vi "Configure Component Values.vi"(0 "VISA resource name":refnum<visa-resource-name>, 1 "Relative Phase":bool, 5 "Frequency (10.000000 MHz)":dbl=10.0, 7 "Unit (MHz)":u16(ring)=1 items=["GHz", "MHz", "KHz", "Hz"], 9 "Phase (0°)":i32, 11 "error in (no error)":errorcluster) -> (4 "VISA resource name out":refnum<visa-resource-name>, 15 "error out":errorcluster)   [LabVIEW 2013, in "Stanford Research CG635.lvlib"]
doc: "Configures the <b>frequency</b> and the <b>phase</b> components to the specified values. \n\n<b>Ranges</b>\nFrequency: 1 µHz to 2.05 GHz\nPhase: -720° to 720°"
uses:
  <instrlib>/Stanford Research CG635/Stanford Research CG635.lvlib
panel:
  # "Note: Set's the current Phase to be a new realtive 0°"
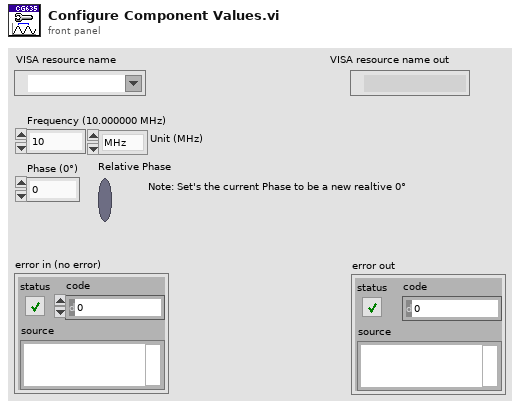
[diagram p1: front panel]
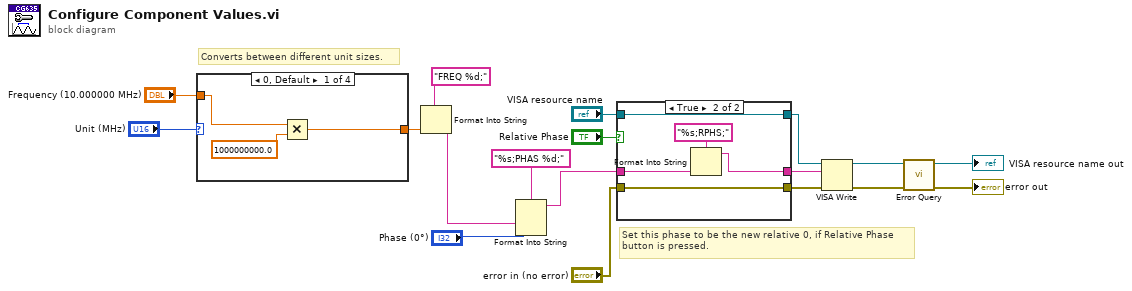
[diagram p0: block diagram]
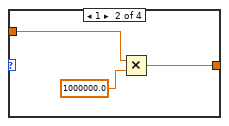
[diagram p3: hidden frame]
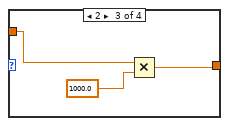
[diagram p4: hidden frame]
diagram:
  # "Set this phase to be the new relative 0, if Relative Phase \nbutton is pressed."
  # "Converts between different unit sizes."
  n1 = case shown="0, Default" "Unit (MHz)" {
    tunnel: "Frequency (10.000000 MHz)" -> [w21 w23 w25 w28]
    tunnel: [w19 w22 w26 w28] -> w13
    frame 0, Default {
      n2 = Multiply(x=w21, y=1000000000.0) -> (x*y=w19:dbl)
    }
    frame 1 {
      n3 = Multiply(x=w23, y=1000000.0) -> (x*y=w22:dbl)
    }
    frame 2 {
      n4 = Multiply(x=w25, y=1000.0) -> (x*y=w26:dbl)
    }
    frame 3 {
    }
  }
  n5 = Format Into String(format string="FREQ %d;", w13) -> (resulting string=w11:string)  [unwired: 2 in, 1 out]
  n6 = Format Into String(format string="%s;PHAS %d;", w11, "Phase (0°)") -> (resulting string=w8:string)  [unwired: 2 in, 1 out]
  n7 = case shown="True" "Relative Phase" {
    tunnel: [w29 w35] -> w12
    tunnel: w8 -> [w29 w34]
    tunnel: "VISA resource name" -> [w31 w33]
    tunnel: [w31 w33] -> w9
    tunnel: "error in (no error)" -> [w30 w32]
    tunnel: [w30 w32] -> w6
    frame False {
    }
    frame True {
      n8 = Format Into String(format string="%s;RPHS;", w34) -> (resulting string=w35:string)  [unwired: 2 in, 1 out]
    }
  }
  n9 = VISA Write(VISA resource name=w9, write buffer=w12, error in (no error)=w6) -> (VISA resource name out=w4:refnum<visa-resource-name>, error out=w3:errorcluster)  [unwired: 1 out]
  n10 = call <instrlib>:"Error Query.vi"("error in (no error)"=w3, "VISA resource name"=w4) -> ("error out"=→"error out":errorcluster, "VISA resource name out"=→"VISA resource name out":refnum<visa-resource-name>)  [unwired: 6 in, 2 out]
